vi "FanPressure.vi"() -> ()   [LabVIEW 2024]
uses:
  <vilib>/drjdpowell/SQLite Library/SQL Connection/Connection.lvclass
  <vilib>/Instr/_visa.llb/VISA Find Search Mode.ctl
  <vilib>/drjdpowell/SQLite Library/SQL Connection/Open (path).vi
  <vilib>/Analysis/baseanly.llb/Mean (DBL).vi
  <vilib>/drjdpowell/SQLite Library/SQL Connection/Open (string).vi
  <vilib>/Instr/_visa.llb/VISA Configure Serial Port (Instr).vi
  <vilib>/drjdpowell/SQLite Library/SQL Connection/Execute SQL (No results).vi
  <vilib>/AdvancedString/Path To Command Line String.vi
  <vilib>/Analysis/NI_AALBase.lvlib
  <vilib>/drjdpowell/SQLite Library/SQLite.lvlib
panel:
  out "user event out":refnum<user-event>
  out "Table Name":string
  in  "Message":string
  out "Table Created":bool
  out "time string":string
  out "date string":string
  out "SQLite Connection":refnum<class "Connection.lvclass">
  in  "View Data":bool
  in  "Reset Plot":bool
  out "Waveform Chart":sgl[][](graph)
  in  "Write To Database":bool
  in  "Interval Time":u32=200
  out "Receive Type":T1
  out "output pwm":dbl
  out "Fan Speed":i32
  out "Fan Shunt Voltage":u16
  out "Fan Power":sgl
  out "Fan current":sgl
  out "Fan Voltage":sgl
  in  "Speed Control":enum32{"Values", "Paramters"}(tab)
  in  "Control Mode":enum32{"", "Radio Selection 2"}(radio)
  in  "Speed Setup":u16=2000 min=10 max=36 step=1
  in  "Output":sgl(knob) min=0 max=1 step=0.001 scale=0.0..1.0 scale format="%.2f"
  in  "Parameter Read Button":bool
  in  "Parameter Write Button":bool
  in  "Fan Speed At Full Output":sgl
  in  "Fan Speed At 50% Output":sgl
  in  "KD":sgl
  in  "KI":sgl=0.001
  in  "KP":sgl=0.002
  in  "DC Power Source Panel":enum32{"Page 1", "Page 2"}(tab)
  out "Current Output (A)":sgl min=10 max=36 step=0.1 format="%#_6f"
  out "Voltage Output (V)":sgl min=10 max=36 step=0.1 format="%#_5f"
  in  "Set Voltage (V)":sgl=15.0 min=10 max=36 step=0.1 format="%#.4f"
  in  "Write Data":bool
  in  "Start Button":bool
  out "Connected?":bool
  out "Serial Port":refnum<visa-resource-name>
  in  "stop":bool
  in  "Tab Control":enum32{"Readings", "Raw Data"}(tab)
  out "Waveform Chart 2":dbl[][](graph)
  out "data":dynamicdata(graph) caption="Raw Data"
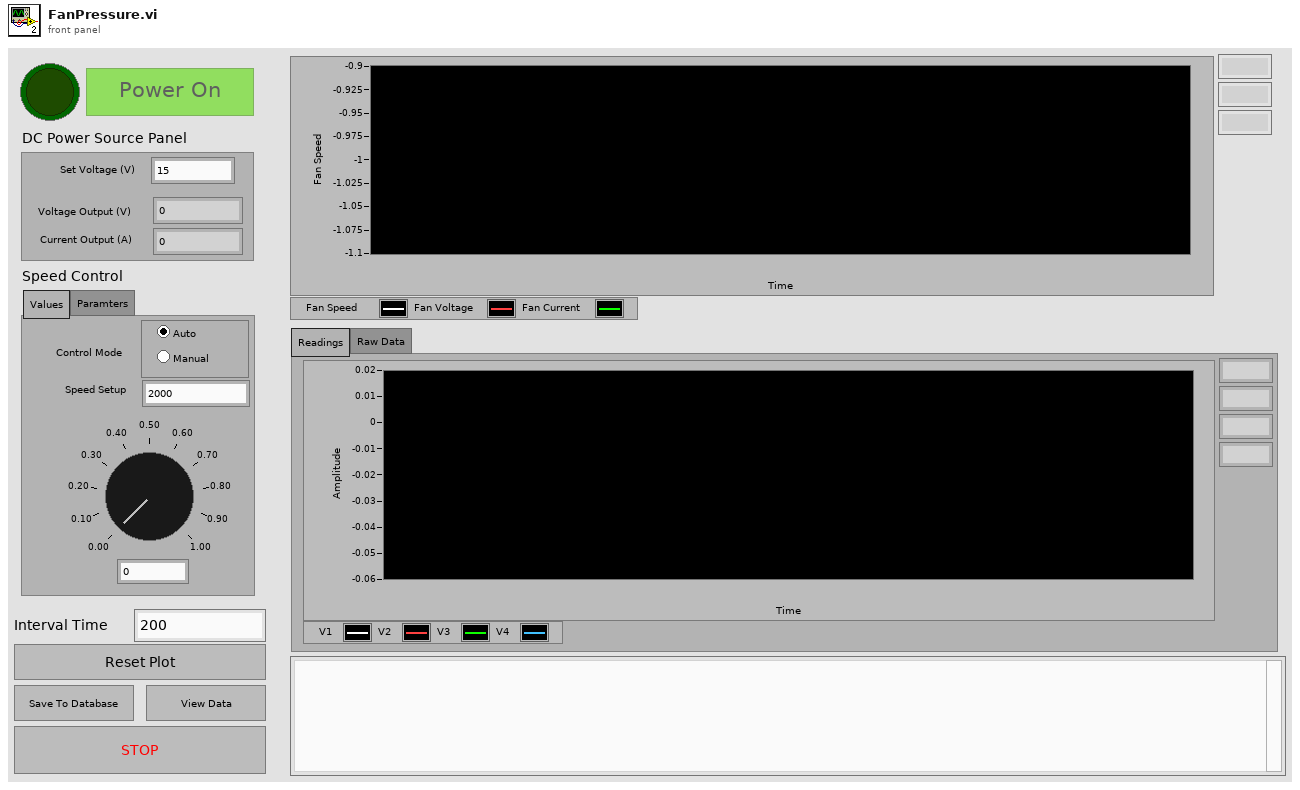
[diagram p1: front panel]
types:
  T1 = cluster{u8, u8, u8, u8, u16, u16, i16, i16, i16, i16, u16, u16, u16, u16, u16, u16, u8, u8, u8, u8}
  T2 = enum16{"New or existing", "Existing", "Read only"}
  T3 = enum8{"Enabled", "Disabled", "Disabled and Grayed Out"}
  T4 = enum32{"Invalid", "Standard", "Closed", "Hidden", "Minimized", "Maximized"}
  T5 = cluster{u32, "Fan current":sgl, "Fan current":sgl, "Fan current":sgl, "Fan Power":sgl, sgl, sgl, sgl, sgl, sgl, "Current Output (A)":sgl, "Voltage Output (V)":sgl}
  T6 = enum16{"big-endian, network order", "native, host order", "little-endian"}
  T7 = typedef "VISA Find Search Mode.ctl" = u32
  T8 = cluster{"y":u8, "y":u8, "y":u8, u8, u16, "Speed Setup":u16, u16, u16, "y":u8, "y":u8, "y":u8, "y":u8}
  T9 = cluster{"y":u8, "y":u8, "y":u8, "y":u8, "KP":sgl, "KI":sgl, "KD":sgl, "Fan Speed At 50% Output":sgl, "Fan Speed At Full Output":sgl, "y":u8, "y":u8, "y":u8, "y":u8}
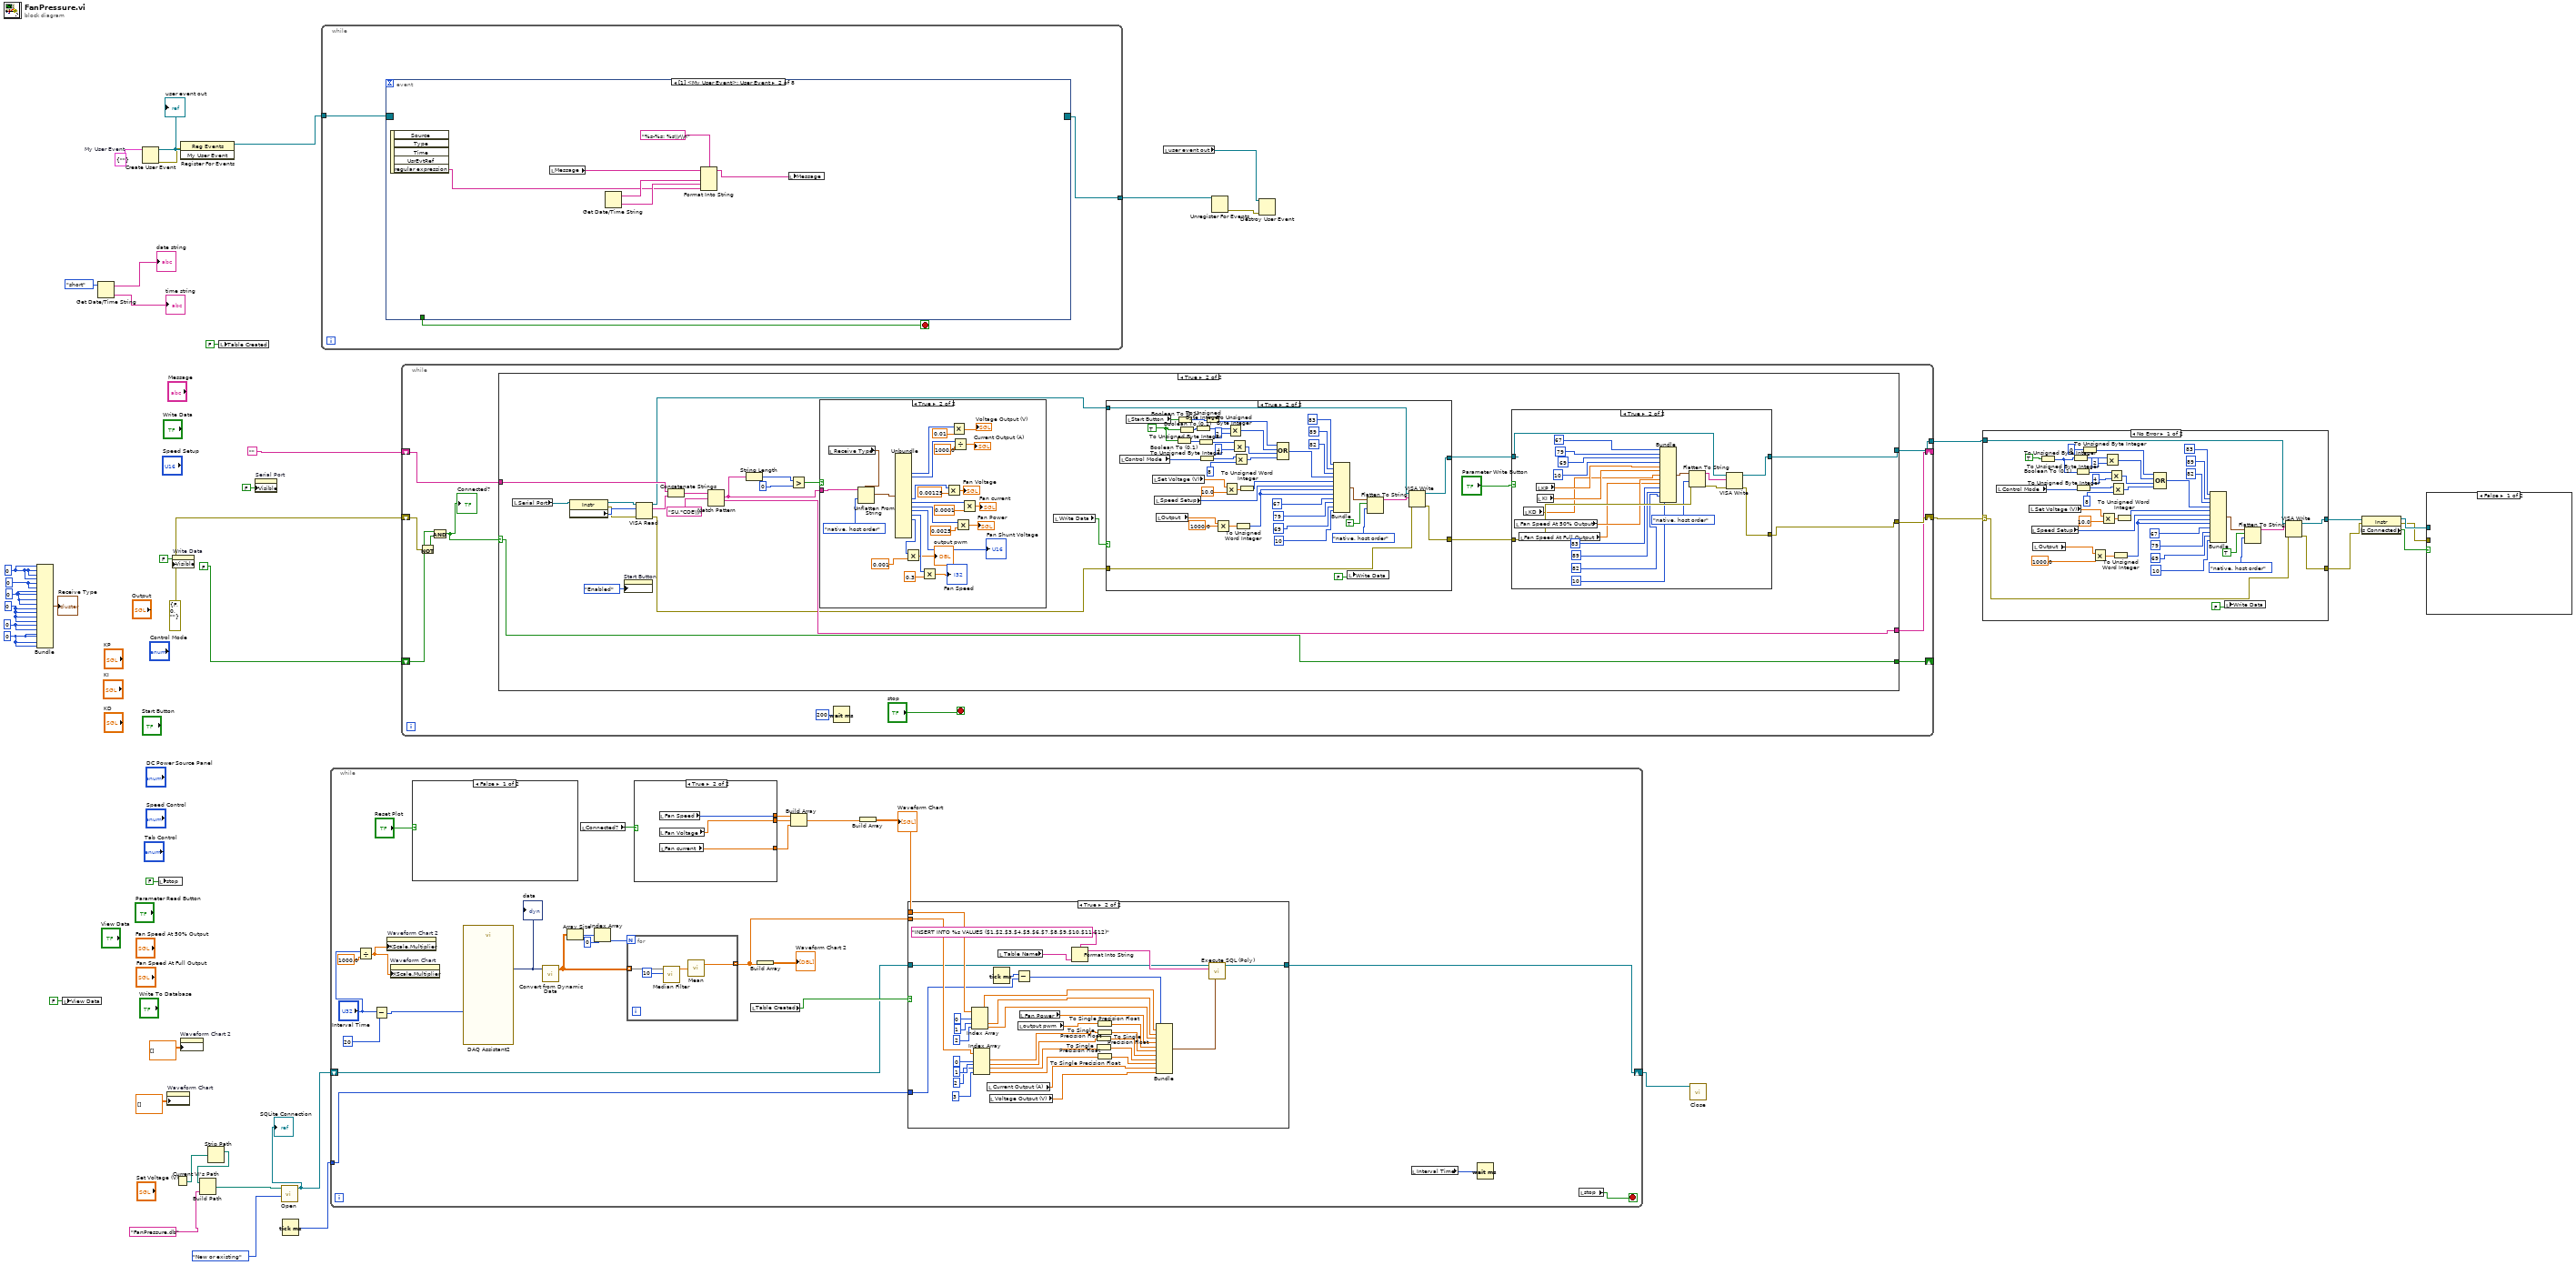
[diagram p0: block diagram]
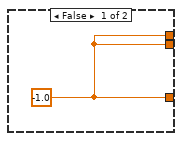
[diagram p3: hidden frame]
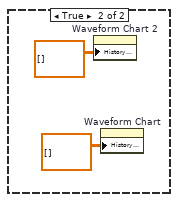
[diagram p4: hidden frame]
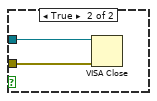
[diagram p5: hidden frame]
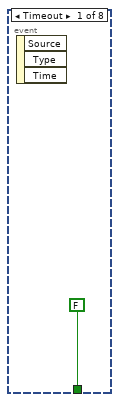
[diagram p7: hidden frame]
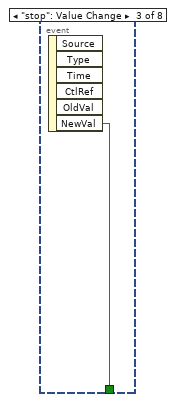
[diagram p8: hidden frame]
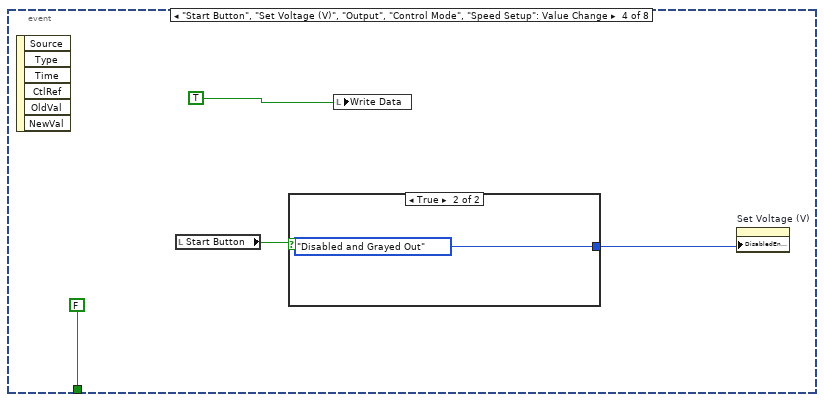
[diagram p9: hidden frame]
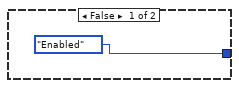
[diagram p10: hidden frame]
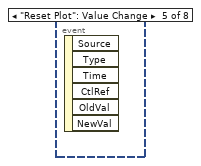
[diagram p11: hidden frame]
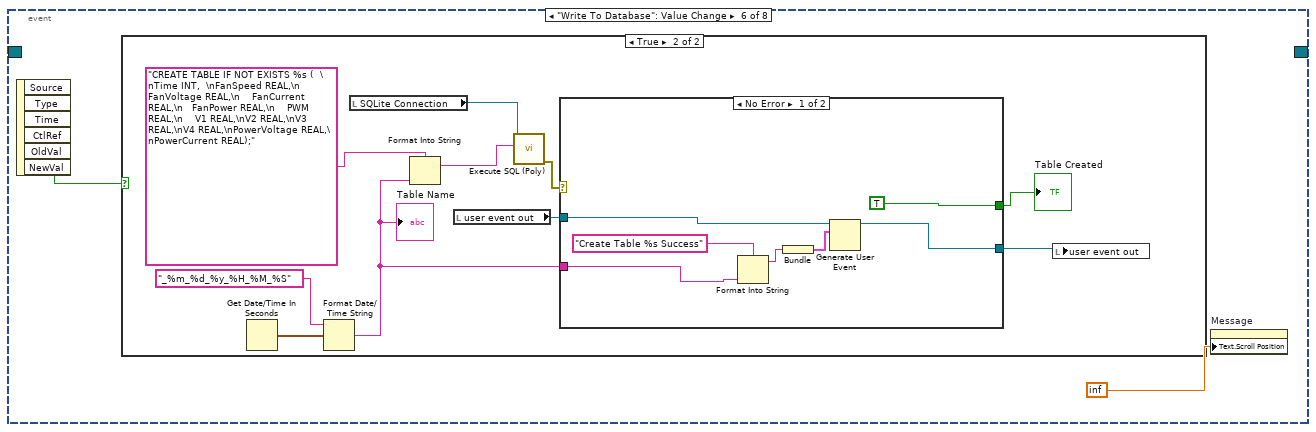
[diagram p12: hidden frame]
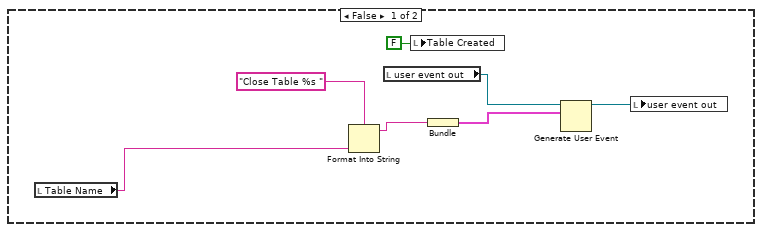
[diagram p13: hidden frame]
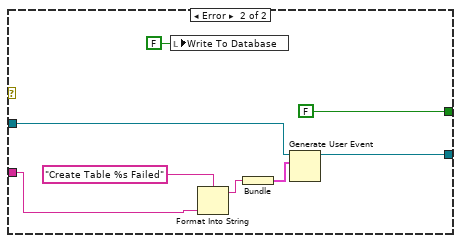
[diagram p14: hidden frame]
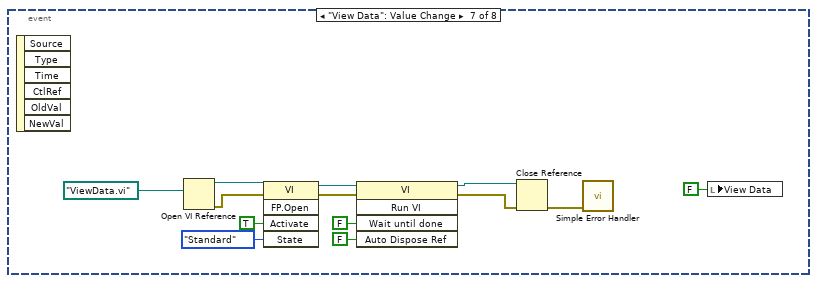
[diagram p15: hidden frame]
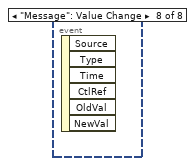
[diagram p16: hidden frame]
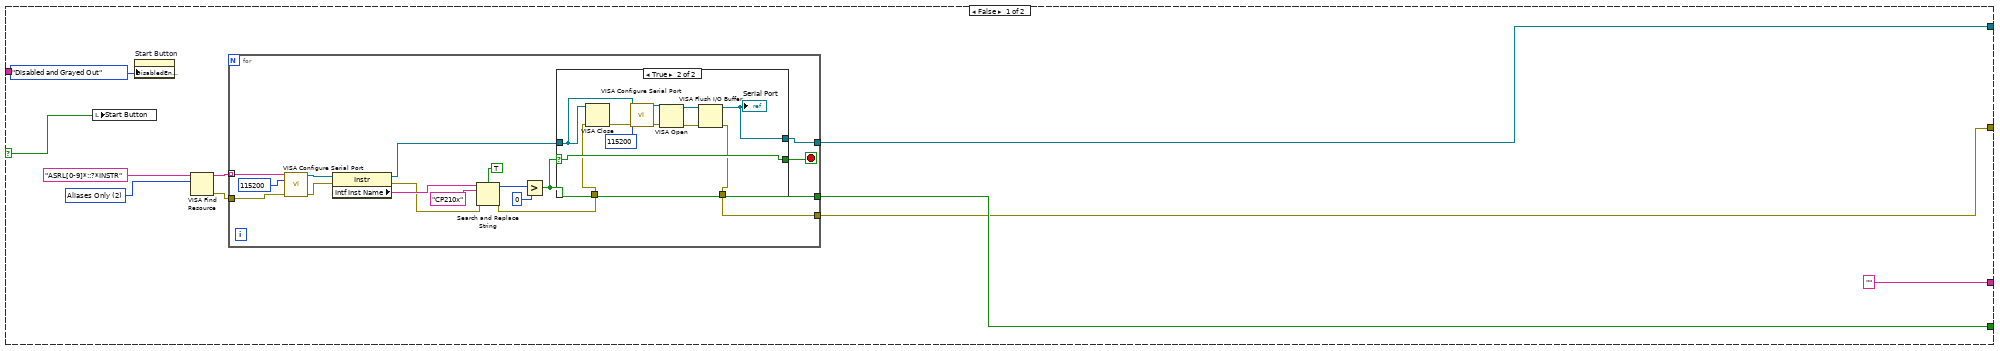
[diagram p17: hidden frame]
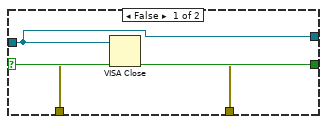
[diagram p18: hidden frame]
diagram:
  w16 = cluster{"regular expression":string} {"regular expression"=""}  # My User Event
  w33 = u16 0
  w35 = u8 0
  w36 = i16 0
  w34 = u16 0
  w37 = u16 0
  w38 = u8 0
  n1 = Bundle(w38, w38, w38, w38, w37, w37, w36, w36, w36, w36, w33, w33, w33, w33, w34, w34, w35, w35, w35, w35) -> (→"Receive Type":T1)  [unwired: 1 in]
  n2 = local write "View Data"(FALSE ("View Data")) -> ()
  n3 = Get Date/Time String(date format (0)=enum16{"short", "long", "abbreviated"}."short") -> (date string=→"date string":string, time string=→"time string":string)  [unwired: 2 in]
  n4 = Create User Event(user event datatype=w16) -> (user event=w15:refnum<user-event>, error out=w13:errorcluster)  [unwired: 1 in]
  "user event out" <- w15
  n5 = local write "stop"(FALSE ("stop")) -> ()
  n6 = property on="Waveform Chart" class="WFChart (strict)"("History Data"=dbl[][] []) -> ()  [unwired: 2 in, 2 out]
  n7 = property on="Write Data" class="Bool (strict)"("Visible"=FALSE) -> ()  [unwired: 2 in, 2 out]
  n8 = Current VI's Path() -> (path=w7:path)
  n9 = property on="Waveform Chart 2" class="WFChart (strict)"("History Data"=dbl[][] []) -> ()  [unwired: 2 in, 2 out]
  n10 = register-events(error in=w13, w15) -> (reference out=w14:refnum<event-registration>)  [unwired: 1 in, 1 out]
  n11 = Strip Path(path=w7) -> (stripped path=w6:path)  [unwired: 1 out]
  n12 = Build Path(base path=w6, name or relative path="FanPressure.db" ("db file")) -> (appended path=w8:path)
  n13 = local write "Table Created"(FALSE ("Table Created")) -> ()
  n14 = property on="Serial Port" class="VISAName"("Visible"=FALSE) -> ()  [unwired: 2 in, 2 out]
  n15 = call-poly <vilib>:"Open.vi"("File Option"=T2."New or existing", "db file"=w8) -> ("SQLite Connection"=w5:refnum<class "Connection.lvclass">)  [unwired: 8 in, 1 out]
  "SQLite Connection" <- w5
  n16 = Tick Count (ms)() -> (millisecond timer value=w2:u32)
  n17 = while {
    tunnel: w14 -> [w44]
    tunnel: [w43] -> w12
    stop <- w45 stop-if-true
    n18 = event shown="[1] <My User Event>: User Event" {
      selector: w44 -> [_ _ _ _ _ _ _ _]
      dyn-events: [_ _ _ _ _ _ _ _] -> w43
      timeout: _ -> [_ _ _ _ _ _ _ _]
      tunnel: [FALSE ("NewVal") _ w53 FALSE ("NewVal") _ _ _ _] -> w45
      event Timeout {
        n19 = event-data() -> ()  [unwired: 1 in, 3 out]
      }
      event User Event {
        n20 = event-data() -> ("regular expression"=w47:string)  [unwired: 1 in, 4 out]
        n21 = local read "Message"() -> (w52:string)
        n22 = Get Date/Time String() -> (date string=w51:string, time string=w50:string)  [unwired: 3 in]
        n23 = Format Into String(format string="%s-%s: %s\\r\\n", initial string=w52, w51, w50, w47) -> (resulting string=w49:string)  [unwired: 1 in, 1 out]
        n24 = local write "Message"(w49) -> ()
      }
      event "stop": Value Change {
        n25 = event-data() -> ("NewVal"=w53:bool)  [unwired: 1 in, 5 out]
      }
      event "Start Button", "Set Voltage (V)", "Output", "Control Mode", "Speed Setup": Value Change {
        n26 = event-data() -> ()  [unwired: 1 in, 6 out]
        n27 = local read "Start Button"() -> (w55:bool)
        n28 = case shown="True" w55 {
          tunnel: [T3."Enabled" ("Disabled") T3."Disabled and Grayed Out" ("Disabled")] -> w54
          frame False {
          }
          frame True {
          }
        }
        n29 = local write "Write Data"(TRUE ("Write Data")) -> ()
        n30 = property on="Set Voltage (V)" class="DigNum (strict)"("DisabledEnum"=w54) -> ()  [unwired: 2 in, 2 out]
      }
      event "Reset Plot": Value Change {
        n31 = event-data() -> ()  [unwired: 1 in, 6 out]
      }
      event "Write To Database": Value Change {
        n32 = event-data() -> ("NewVal"=w61:bool)  [unwired: 1 in, 5 out]
        n33 = case shown="True" w61 {
          frame False {
            n34 = local read "Table Name"() -> (w67:string)
            n35 = Format Into String(format string="Close Table %s ", w67) -> (resulting string=w64:string)  [unwired: 2 in, 1 out]
            n36 = local read "user event out"() -> (w65:refnum<user-event>)
            n37 = local write "Table Created"(FALSE ("Table Created")) -> ()
            n38 = Bundle(w64) -> (w63:cluster{string})  [unwired: 1 in]
            n39 = Generate User Event(user event=w65, event data cluster=w63) -> (user event out=w62:refnum<user-event>)  [unwired: 2 in, 1 out]
            n40 = local write "user event out"(w62) -> ()
          }
          frame True {
            n41 = Get Date/Time In Seconds() -> (seconds since 1Jan1904=w77:timestamp)
            n42 = Format Date/Time String(time format string (%c)="_%m_%d_%y_%H_%M_%S", seconds (now)=w77) -> (date/time string=w69:string)  [unwired: 1 in]
            "Table Name" <- w69
            n43 = local read "SQLite Connection"() -> (w78:refnum<class "Connection.lvclass">)
            n44 = Format Into String(format string="CREATE TABLE IF NOT EXISTS %s (  \nTime INT,  \nFanSpeed REAL,\n    FanVoltage REAL,\n    FanCurrent REAL,\n   FanPower REAL,\n    PWM REAL,\n    V1 REAL,\nV2 REAL,\nV3 REAL,\nV4 REAL,\nPowerVoltage REAL,\nPowerCurrent REAL);" ("SQL"), w69) -> (resulting string=w74:string)  [unwired: 2 in, 1 out]
            n45 = local read "user event out"() -> (w71:refnum<user-event>)
            n46 = call-poly <vilib>:"Execute SQL (Poly).vi"("SQL"=w74, "SQLite Connection in"=w78) -> ("error out"=w73:errorcluster)  [unwired: 8 in, 1 out]
            n47 = case shown="No Error" w73 {
              tunnel: [TRUE ("Table Created") FALSE ("Table Created")] -> w72
              tunnel: w71 -> [w79 w88]
              tunnel: [w80 w87] -> w70
              tunnel: w69 -> [w81 w86]
              frame No Error {
                n48 = Format Into String(format string="Create Table %s Success", w81) -> (resulting string=w84:string)  [unwired: 2 in, 1 out]
                n49 = Bundle(w84) -> (w83:cluster{string})  [unwired: 1 in]
                n50 = Generate User Event(user event=w79, event data cluster=w83) -> (user event out=w80:refnum<user-event>)  [unwired: 2 in, 1 out]
              }
              frame Error {
                n51 = local write "Write To Database"(FALSE ("Write To Database")) -> ()
                n52 = Format Into String(format string="Create Table %s Failed", w86) -> (resulting string=w91:string)  [unwired: 2 in, 1 out]
                n53 = Bundle(w91) -> (w90:cluster{string})  [unwired: 1 in]
                n54 = Generate User Event(user event=w88, event data cluster=w90) -> (user event out=w87:refnum<user-event>)  [unwired: 2 in, 1 out]
              }
            }
            "Table Created" <- w72
            n55 = local write "user event out"(w70) -> ()
          }
        }
        n56 = property on="Message" class="Str"("Text.Scroll Position"=inf) -> ()  [unwired: 2 in, 2 out]
      }
      event "View Data": Value Change {
        n57 = event-data() -> ()  [unwired: 1 in, 6 out]
        n58 = Open VI Reference(vi path=path "ViewData.vi") -> (vi reference=w104:refnum<vi>, error out=w97:errorcluster)  [unwired: 5 in]
        n59 = invoke class="VI" method="FP.Open"(reference=w104, error in=w97, "Activate"=TRUE ("Activate?"), "State"=T4."Standard") -> (reference out=w101:refnum<vi>, error out=w100:errorcluster)  [unwired: 1 in, 3 out]
        n60 = invoke class="VI" method="Run VI"(reference=w101, error in=w100, "Wait until done"=FALSE ("Wait Until Done"), "Auto Dispose Ref"=FALSE ("Auto Dispose Reference")) -> (reference out=w96:refnum<vi>, error out=w95:errorcluster)  [unwired: 1 in, 3 out]
        n61 = Close Reference(reference=w96, error in (no error)=w95) -> (error out=w94:errorcluster)
        n62 = call <vilib>:"Simple Error Handler.vi"("error in (no error)"=w94) -> ()  [unwired: 4 in, 5 out]
        n63 = local write "View Data"(FALSE ("View Data")) -> ()
      }
      event "Message": Value Change {
        n64 = event-data() -> ()  [unwired: 1 in, 6 out]
      }
    }
  }
  n65 = while {
    shift-right: [w109] -> w4
    shift-left: w5 -> [w108]
    tunnel: w2 -> [w107]
    stop <- w131 stop-if-true
    n66 = Divide(x="Interval Time", y=1000.0) -> (x/y=w118:dbl)
    n67 = Subtract(x="Interval Time", y=u32 20) -> (x-y=w127:u32)
    n68 = property on="Waveform Chart 2" class="WFChart (strict)"("XScale.Multiplier"=w118) -> ()  [unwired: 2 in, 2 out]
    n69 = property on="Waveform Chart" class="WFChart (strict)"("XScale.Multiplier"=w118) -> ()  [unwired: 2 in, 2 out]
    n70 = case shown="False" "Reset Plot" {
      frame False {
      }
      frame True {
        n71 = property on="Waveform Chart 2" class="WFChart (strict)"("History Data"=dbl[][] []) -> ()  [unwired: 2 in, 2 out]
        n72 = property on="Waveform Chart" class="WFChart (strict)"("History Data"=dbl[][] []) -> ()  [unwired: 2 in, 2 out]
      }
    }
    n73 = call "DAQ Assistant2"("number of samples"=w127) -> ("data"=w129:dynamicdata)  [unwired: 16 in, 2 out]
    "data" <- w129
    n74 = call "Convert from Dynamic Data"("Dynamic Data Type"=w129) -> ("Array"=w126:dbl[][])  [unwired: 3 in]
    n75 = Array Size(array=w126) -> (size(s)=w125:i32[])
    n76 = local read "Connected?"() -> (w117:bool)
    n77 = Index Array(array=w125, index=0) -> (element=w123:i32)
    n78 = for {
      N: w123 -> [_]
      tunnel: w126 -> [w176] mode=indexing
      tunnel: [w173] -> w112 mode=indexing
      n79 = call <vilib>:"Median Filter.vi"("left rank"=10, "X"=w176) -> ("Filtered X"=w174:dbl[])  [unwired: 8 in, 1 out]
      n80 = call-poly <vilib>:"Mean.vi"("X"=w174) -> ("mean"=w173:dbl)  [unwired: 1 out]
    }
    n81 = case shown="True" w117 {
      tunnel: [w167 w170] -> w116
      tunnel: [w167 w169] -> w115
      tunnel: [w167 w168] -> w114
      frame False {
        w167 = sgl -1.0 ("Fan current")
      }
      frame True {
        n82 = local read "Fan Speed"() -> (w168:i32)
        n83 = local read "Fan Voltage"() -> (w169:sgl)
        n84 = local read "Fan current"() -> (w170:sgl)
      }
    }
    n85 = local read "Table Created"() -> (w110:bool)
    n86 = Build Array(w112) -> (→"Waveform Chart 2":dbl[][])
    n87 = Build Array(w114, w115, w116) -> (w111:sgl[])
    n88 = Build Array(w111) -> (→"Waveform Chart":sgl[][])
    n89 = case shown="True" w110 {
      tunnel: w112 -> [_ w162]
      tunnel: w111 -> [_ w166]
      tunnel: w108 -> [w132 w147]
      tunnel: [w132 w146] -> w109
      tunnel: w107 -> [_ w134]
      frame False {
      }
      frame True {
        n90 = Index Array(array=w166, index #1=0 ("index"), index #2=1 ("index"), index #3=2 ("index")) -> (element #1=w157:sgl, element #2=w156:sgl, element #3=w155:sgl)
        n91 = Index Array(array=w162, index #1=0 ("index"), index #2=1 ("index"), index #3=2 ("index"), index #4=3 ("index")) -> (element #1=w139:dbl, element #2=w141:dbl, element #3=w143:dbl, element #4=w145:dbl)
        n92 = local read "Current Output (A)"() -> (w153:sgl)
        n93 = local read "Voltage Output (V)"() -> (w152:sgl)
        n94 = Tick Count (ms)() -> (millisecond timer value=w135:u32)
        n95 = local read "Table Name"() -> (w149:string)
        n96 = Subtract(x=w135, y=w134) -> (x-y=w133:u32)
        n97 = local read "output pwm"() -> (w137:dbl)
        n98 = local read "Fan Power"() -> (w154:sgl)
        n99 = Format Into String(format string="INSERT INTO %s VALUES ($1,$2,$3,$4,$5,$6,$7,$8,$9,$10,$11,$12)" ("SQL"), w149) -> (resulting string=w148:string)  [unwired: 2 in, 1 out]
        n100 = To Single Precision Float(number=w141) -> (single precision float=w140:sgl)
        n101 = To Single Precision Float(number=w143) -> (single precision float=w142:sgl)
        n102 = To Single Precision Float(number=w137) -> (single precision float=w136:sgl)
        n103 = To Single Precision Float(number=w139) -> (single precision float=w138:sgl)
        n104 = To Single Precision Float(number=w145) -> (single precision float=w144:sgl)
        n105 = Bundle(w133, "Fan current"=w157, "Fan current"=w156, "Fan current"=w155, "Fan Power"=w154, w136, w138, w140, w142, w144, "Current Output (A)"=w153, "Voltage Output (V)"=w152) -> (w151:T5)  [unwired: 1 in]
        n106 = call-poly <vilib>:"Execute SQL (Poly).vi"("Parameter(s)"=w151, "SQL"=w148, "SQLite Connection in"=w147) -> ("SQLite Connection"=w146:refnum<class "Connection.lvclass">)  [unwired: 7 in, 1 out]
      }
    }
    n107 = local read "Interval Time"() -> (w130:u32)
    n108 = Wait (ms)(milliseconds to wait=w130) -> ()  [unwired: 1 out]
    n109 = local read "stop"() -> (w131:bool)
  }
  n110 = while {
    shift-right: [w186] -> _
    shift-left: FALSE -> [w184]
    shift-right: [w185] -> w29
    shift-left: errorcluster {"status"=FALSE, "code"=0, "source"=""} ("error in (no error)") -> [w180]
    tunnel: [w182] -> w30
    shift-right: [w179] -> _
    shift-left: "" -> [w178]
    stop <- "stop" stop-if-true
    n111 = Not(x=w180) -> (.not. x?=w183:bool)
    n112 = And(x=w184, y=w183) -> (x .and. y?=w177:bool)
    "Connected?" <- w177
    n113 = case shown="True" w177 {
      selector: w177 -> [w189 w238]
      tunnel: [w193 w238] -> w186
      tunnel: [w192 w231] -> w185
      tunnel: [w191 w233] -> w182
      tunnel: w178 -> [_ w247]
      tunnel: ["" w244] -> w179
      frame False {
        w196 = T7 2 items=["Canonical Names Only"=0, "Aliases Only"=2, "Include Matching Aliases"=3, "Include All Aliases"=4] ("Search Mode")
        n114 = local write "Start Button"(w189) -> ()
        n115 = property on="Start Button" class="Bool (strict)"("DisabledEnum"=T3."Disabled and Grayed Out" ("Disabled")) -> ()  [unwired: 2 in, 2 out]
        n116 = VISA Find Resource(10:w196, 11:"ASRL[0-9]*::?*INSTR" ("expression (\"?*\")")) -> (0:w194:errorcluster, 3:w195:string[])  [unwired: 1 in, 1 out]
        n117 = for {
          tunnel: w195 -> [w202] mode=indexing
          tunnel: w194 -> [w214]
          tunnel: [w206] -> w193
          tunnel: [w199] -> w192
          tunnel: [w198] -> w191
          stop <- w205 stop-if-true
          n118 = call-poly "VISA Configure Serial Port"("VISA resource name"=w202, "baud rate (9600)"=u32 115200, "error in (no error)"=w214) -> ("VISA resource name out"=w201:refnum<visa-resource-name>, "error out"=w213:errorcluster)  [unwired: 11 in]
          n119 = property class="Instr"(reference=w201, error in=w213) -> (reference out=w204:refnum<visa-resource-name>, error out=w210:errorcluster, "Intf Inst Name"=w212:string)
          n120 = Search and Replace String(case sensitive?=TRUE ("ignore case? (F)"), input string=w212, search string="CP210x", error in=w210) -> (number of replacements=w208:i32, error out=w200:errorcluster)  [unwired: 4 in, 2 out]
          n121 = Greater?(x=w208, y=0) -> (0:w206:bool)
          n122 = case shown="True" w206 {
            selector: w206 -> [w218 w229]
            tunnel: [w218 w229] -> w205
            tunnel: w204 -> [w215 w227]
            tunnel: w200 -> [w217 w228]
            tunnel: [w216 w221] -> w199
            tunnel: [w215 w223] -> w198
            frame False {
              n123 = VISA Close(VISA resource name=w215, error in (no error)=w217) -> (error out=w216:errorcluster)
            }
            frame True {
              n124 = VISA Close(VISA resource name=w227, error in (no error)=w228) -> (error out=w220:errorcluster)
              n125 = call-poly "VISA Configure Serial Port"("VISA resource name"=w227, "baud rate (9600)"=u32 115200, "error in (no error)"=w220) -> ("VISA resource name out"=w225:refnum<visa-resource-name>, "error out"=w219:errorcluster)  [unwired: 11 in]
              n126 = VISA Open(error in (no error)=w219, VISA resource name=w225) -> (VISA resource name=w224:refnum<visa-resource-name>, error out=w222:errorcluster)  [unwired: 3 in]
              n127 = VISA Flush I/O Buffer(VISA resource name=w224, error in (no error)=w222) -> (VISA resource name out=w223:refnum<visa-resource-name>, error out=w221:errorcluster)  [unwired: 1 in]
              "Serial Port" <- w223
            }
          }
        }
      }
      frame True {
        n128 = local read "Serial Port"() -> (w252:refnum<visa-resource-name>)
        n129 = property class="Instr"(reference=w252) -> (reference out=w250:refnum<visa-resource-name>, error out=w249:errorcluster, "Serial Settings:Number of Bytes at Serial Port"=w251:u32)  [unwired: 1 in]
        n130 = property on="Start Button" class="Bool (strict)"("DisabledEnum"=T3."Enabled" ("Disabled")) -> ()  [unwired: 2 in, 2 out]
        n131 = VISA Read(VISA resource name=w250, byte count=w251, error in (no error)=w249) -> (VISA resource name out=w239:refnum<visa-resource-name>, read buffer=w248:string, error out=w235:errorcluster)  [unwired: 1 out]
        n132 = Concatenate Strings(w247, w248) -> (w245:string)
        n133 = Match Pattern(string=w245, regular expression="SU.*COE\\n") -> (match substring=w243:string, after substring=w244:string)  [unwired: 1 in, 2 out]
        n134 = String Length(string=w243) -> (length=w242:i32)
        n135 = Greater?(x=w242, y=0) -> (0:w240:bool)
        n136 = case shown="True" w240 {
          tunnel: w243 -> [_ w345]
          frame False {
          }
          frame True {
            n137 = local read "Receive Type"() -> (w320:T1)
            n138 = Unflatten From String(type=w320, binary string=w345, byte order (0:big-endian, network order)=T6."native, host order") -> (value=w343:T1)  [unwired: 2 in, 2 out]
            n139 = Unbundle(w343) -> (w342:u16, w338:u16, w335:u16, w331:u16, w329:u16, →"Fan Shunt Voltage":u16, w325:u16, w323:u16)  [unwired: 12 out]
            n140 = Multiply(x=w323, y=0.001) -> (x*y=→"output pwm":dbl)
            n141 = Multiply(x=w325, y=0.3) -> (x*y=→"Fan Speed":dbl)
            n142 = Multiply(x=w335, y=0.00125) -> (x*y=→"Fan Voltage":dbl)
            n143 = Multiply(x=w342, y=0.01) -> (x*y=→"Voltage Output (V)":dbl)
            n144 = Divide(x=w338, y=1000.0) -> (x/y=→"Current Output (A)":dbl)
            n145 = Multiply(x=w329, y=0.0025) -> (x*y=→"Fan Power":dbl)
            n146 = Multiply(x=w331, y=0.0001) -> (x*y=→"Fan current":dbl)
          }
        }
        n147 = local read "Write Data"() -> (w236:bool)
        n148 = case shown="True" w236 {
          tunnel: w239 -> [w277 w319]
          tunnel: [w277 w318] -> w234
          tunnel: w235 -> [w276 w317]
          tunnel: [w276 w316] -> w232
          frame False {
          }
          frame True {
            w278 = TRUE ("Boolean")
            n149 = local read "Control Mode"() -> (w279:enum32{"", "Radio Selection 2"})
            n150 = local read "Start Button"() -> (w312:bool)
            n151 = local read "Set Voltage (V)"() -> (w311:sgl)
            n152 = local read "Speed Setup"() -> (w293:u16)
            n153 = local read "Output"() -> (w291:sgl)
            n154 = Boolean To (0,1)(Boolean=w278) -> (0, 1=w308:i16)
            n155 = Boolean To (0,1)(Boolean=w312) -> (0, 1=w313:i16)
            n156 = Boolean To (0,1)(Boolean=w278) -> (0, 1=w314:i16)
            n157 = To Unsigned Byte Integer(number=w314) -> (unsigned 8bit integer=w303:u8)
            n158 = To Unsigned Byte Integer(number=w308) -> (unsigned 8bit integer=w300:u8)
            n159 = To Unsigned Byte Integer(number=w279) -> (unsigned 8bit integer=w299:u8)
            n160 = To Unsigned Byte Integer(number=w313) -> (unsigned 8bit integer=w307:u8)
            n161 = Multiply(x=w291, y=sgl 1000.0) -> (x*y=w290:sgl)
            n162 = Multiply(x=w311, y=sgl 10.0) -> (x*y=w309:sgl)
            n163 = Multiply(x=w303, y=u8 2) -> (x*y=w301:u8)
            n164 = Multiply(x=w300, y=u8 4) -> (x*y=w295:u8)
            n165 = Multiply(x=w299, y=u8 8 ("x")) -> (x*y=w297:u8)
            n166 = To Unsigned Word Integer(number=w290) -> (unsigned 16bit integer=w289:u16)
            n167 = To Unsigned Word Integer(number=w309) -> (unsigned 16bit integer=w294:u16)
            n168 = Compound Arithmetic op=OR(w307, w301, w295, w297) -> (w306:u8)
            n169 = Bundle("y"=u8 83, "y"=u8 89, "y"=u8 82, w306, w294, "Speed Setup"=w293, w289, w289, "y"=u8 67, "y"=u8 79, "y"=u8 69, "y"=u8 10) -> (w281:T8)  [unwired: 1 in]
            n170 = local write "Write Data"(FALSE ("Write Data")) -> ()
            n171 = Flatten To String(anything=w281, prepend array or string size? (T)=TRUE, byte order (0:big-endian, network order)=T6."native, host order") -> (data string=w280:string)  [unwired: 1 in, 2 out]
            n172 = VISA Write(VISA resource name=w319, write buffer=w280, error in (no error)=w317) -> (VISA resource name out=w318:refnum<visa-resource-name>, error out=w316:errorcluster)  [unwired: 1 out]
          }
        }
        n173 = case shown="True" "Parameter Write Button" {
          tunnel: w234 -> [w254 w275]
          tunnel: [w254 w274] -> w233
          tunnel: w232 -> [w253 w271]
          tunnel: [w253 w272] -> w231
          frame False {
          }
          frame True {
            n174 = local read "Fan Speed At 50% Output"() -> (w263:sgl)
            n175 = local read "Fan Speed At Full Output"() -> (w262:sgl)
            n176 = local read "KD"() -> (w264:sgl)
            n177 = local read "KP"() -> (w266:sgl)
            n178 = local read "KI"() -> (w265:sgl)
            n179 = Bundle("y"=u8 67, "y"=u8 79, "y"=u8 69, "y"=u8 10, "KP"=w266, "KI"=w265, "KD"=w264, "Fan Speed At 50% Output"=w263, "Fan Speed At Full Output"=w262, "y"=u8 83, "y"=u8 89, "y"=u8 82, "y"=u8 10) -> (w257:T9)  [unwired: 1 in]
            n180 = Flatten To String(anything=w257, byte order (0:big-endian, network order)=T6."native, host order", error in (no error)=w271) -> (data string=w255:string, error out=w273:errorcluster)  [unwired: 1 in, 1 out]
            n181 = VISA Write(VISA resource name=w275, write buffer=w255, error in (no error)=w273) -> (VISA resource name out=w274:refnum<visa-resource-name>, error out=w272:errorcluster)  [unwired: 1 out]
          }
        }
      }
    }
    n182 = Wait (ms)(milliseconds to wait=u32 200) -> ()  [unwired: 1 out]
  }
  n183 = local read "user event out"() -> (w10:refnum<user-event>)
  n184 = Unregister For Events(event registration refnum=w12) -> (error out=w11:errorcluster)  [unwired: 1 in]
  n185 = Destroy User Event(user event=w10, error in=w11) -> ()  [unwired: 1 out]
  n186 = call-dynamic "Close.vi"("SQLite Connection in"=w4) -> ()  [unwired: 10 in, 1 out]
  n187 = case shown="No Error" w29 {
    selector: w29 -> [w349 w387]
    tunnel: [w385 w386] -> w27
    tunnel: [w384 w387] -> w26
    tunnel: w30 -> [w348 w386]
    frame No Error {
      n188 = local read "Control Mode"() -> (w350:enum32{"", "Radio Selection 2"})
      n189 = local read "Set Voltage (V)"() -> (w382:sgl)
      n190 = local read "Speed Setup"() -> (w365:u16)
      n191 = local read "Output"() -> (w362:sgl)
      n192 = Boolean To (0,1)(Boolean=TRUE) -> (0, 1=w346:i16)
      n193 = To Unsigned Byte Integer(number=w346) -> (unsigned 8bit integer=w375:u8)
      n194 = To Unsigned Byte Integer(number=w346) -> (unsigned 8bit integer=w372:u8)
      n195 = To Unsigned Byte Integer(number=w350) -> (unsigned 8bit integer=w371:u8)
      n196 = To Unsigned Byte Integer(number=u8 0) -> (unsigned 8bit integer=w379:u8)
      n197 = Multiply(x=w362, y=sgl 1000.0) -> (x*y=w361:sgl)
      n198 = Multiply(x=w382, y=sgl 10.0) -> (x*y=w380:sgl)
      n199 = Multiply(x=w375, y=u8 2) -> (x*y=w373:u8)
      n200 = Multiply(x=w372, y=u8 4) -> (x*y=w367:u8)
      n201 = Multiply(x=w371, y=u8 8 ("x")) -> (x*y=w369:u8)
      n202 = To Unsigned Word Integer(number=w361) -> (unsigned 16bit integer=w360:u16)
      n203 = To Unsigned Word Integer(number=w380) -> (unsigned 16bit integer=w366:u16)
      n204 = Compound Arithmetic op=OR(w379, w373, w367, w369) -> (w378:u8)
      n205 = Bundle("y"=u8 83, "y"=u8 89, "y"=u8 82, w378, w366, "Speed Setup"=w365, w360, w360, "y"=u8 67, "y"=u8 79, "y"=u8 69, "y"=u8 10) -> (w352:T8)  [unwired: 1 in]
      n206 = local write "Write Data"(FALSE ("Write Data")) -> ()
      n207 = Flatten To String(anything=w352, prepend array or string size? (T)=TRUE, byte order (0:big-endian, network order)=T6."native, host order") -> (data string=w351:string)  [unwired: 1 in, 2 out]
      n208 = VISA Write(VISA resource name=w348, write buffer=w351, error in (no error)=w349) -> (VISA resource name out=w385:refnum<visa-resource-name>, error out=w384:errorcluster)  [unwired: 1 out]
    }
    frame Error {
    }
  }
  n209 = property class="Instr"(reference=w27, error in=w26) -> (reference out=w24:refnum<visa-resource-name>, error out=w23:errorcluster, "Is Connected"=w25:bool)
  n210 = case shown="False" w25 {
    tunnel: w24 -> [_ w389]
    tunnel: w23 -> [_ w388]
    frame False {
    }
    frame True {
      n211 = VISA Close(VISA resource name=w389, error in (no error)=w388) -> ()  [unwired: 1 out]
    }
  }
